vi "set_tags.vi"(8 "error in (no error)":errorcluster, 10 "tags":string[](array[string]), 11 "Image.lvclass in":refnum<class "Image.lvclass">) -> (0 "error out":errorcluster, 3 "Image.lvclass out":refnum<class "Image.lvclass">)   [LabVIEW 2010, in "Image.lvclass"]
uses:
  Image.lvclass
  Image.lvclass/Image.ctl
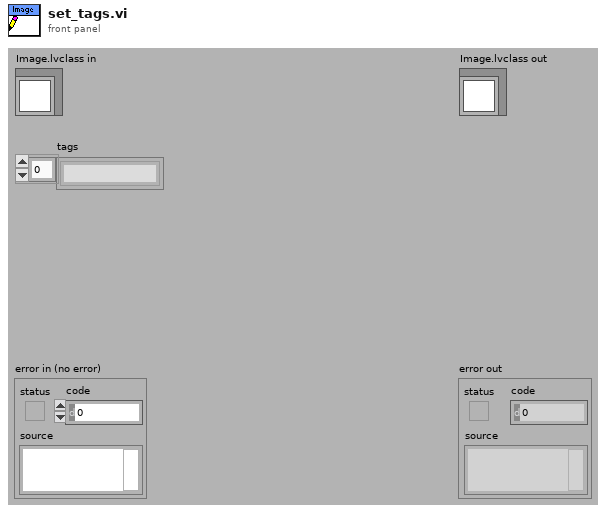
[diagram p1: front panel]
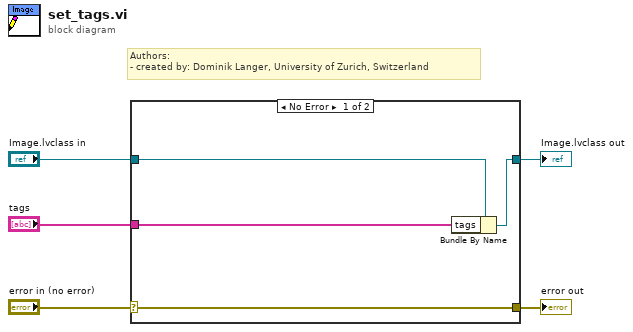
[diagram p0: block diagram]
diagram:
  # "Authors: \n- created by: Dominik Langer, University of Zurich, Switzerland"
  n1 = case shown="No Error" "error in (no error)" {
    selector: "error in (no error)" -> [w9 w10]
    tunnel: [w9 w10] -> w4
    tunnel: [w7 w11] -> w2
    tunnel: "Image.lvclass in" -> [w8 w11]
    tunnel: "tags" -> [w6 _]
    frame No Error {
      n2 = Bundle By Name(cluster=w8, "tags"=w6) -> (w7:refnum<class "Image.lvclass">)
    }
    frame Error {
    }
  }
  "error out" <- w4
  "Image.lvclass out" <- w2
